vi "command_jlink.vi"(0 "user":string, 5 "Device":string, 7 "conection type":string, 9 "speed":string, 11 "uploader_erase?":string) -> (4 "command_jlink":string)   [LabVIEW 2023]
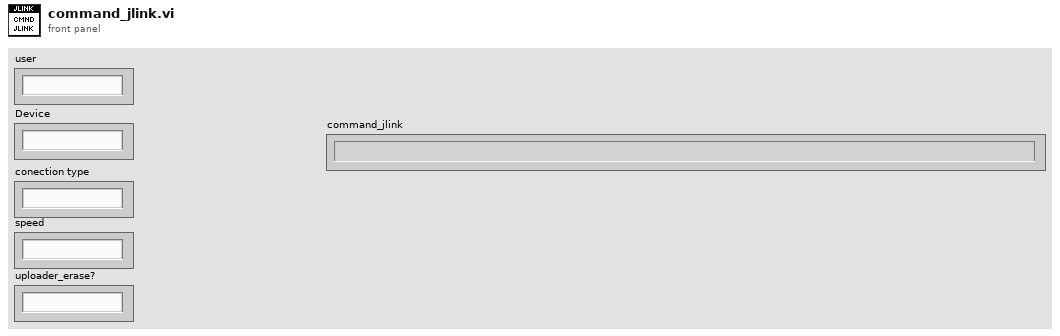
[diagram p1: front panel]
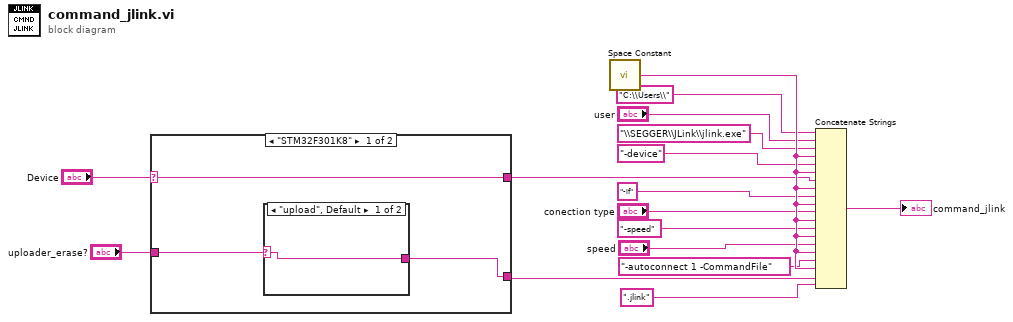
[diagram p0: block diagram]
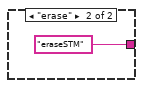
[diagram p2: hidden frame]
diagram:
  n1 = case shown="\"STM32F301K8\"" "Device" {
    selector: "Device" -> [w19 w23]
    tunnel: [w19 w23] -> w5
    tunnel: "uploader_erase?" -> [w18 w22]
    tunnel: [w17 w22] -> w1
    frame "STM32F301K8" {
      n2 = case shown="\"upload\", Default" w18 {
        selector: w18 -> [w20 _]
        tunnel: [w20 "eraseSTM" ("uploader_erase?")] -> w17
        frame "upload", Default {
        }
        frame "erase" {
        }
      }
    }
    frame "Renesas", Default {
    }
  }
  n3 = call <vilib>:"Space Constant.vi"() -> ("String"=w15:string)
  n4 = Concatenate Strings("C:\\Users\\" ("string"), "user", "\\SEGGER\\JLink\\jlink.exe" ("string"), w15, "-device" ("string"), w15, w5, w15, "-if" ("string"), w15, "conection type", w15, "-speed" ("string"), w15, "speed", w15, "-autoconnect 1 -CommandFile" ("string"), w15, w1, ".jlink" ("string")) -> (→"command_jlink":string)
